vi "options dialog.vi"(9 "mode":string, 10 "Args":T1) -> (1 "mode out":string, 2 "Args out":T1)   [LabVIEW 2016]
uses:
  controls/CL Args.ctl
panel:
  in  "-nobdcosm":bool
  in  "-nobdpos":bool
  in  "DONE":bool
  in  "-nobd":bool
  in  "-nofppos":bool
  in  "-nofp":bool
  in  "-noattr":bool
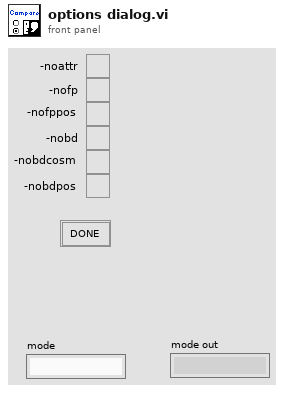
[diagram p1: front panel]
types:
  T1 = typedef "CL Args.ctl" = cluster{"-noattr":bool, "-nofp":bool, "-nofppos":bool, "-nobd":bool, "-nobdcosm":bool, "-nobdpos":bool}
  T2 = enum8{"Enabled", "Disabled", "Disabled and Grayed Out"}
  T3 = enum32{"invalid app kind", "Development System", "Run Time System", "Student Edition", "Embedded LabVIEW", "Evaluation", "Custom"}
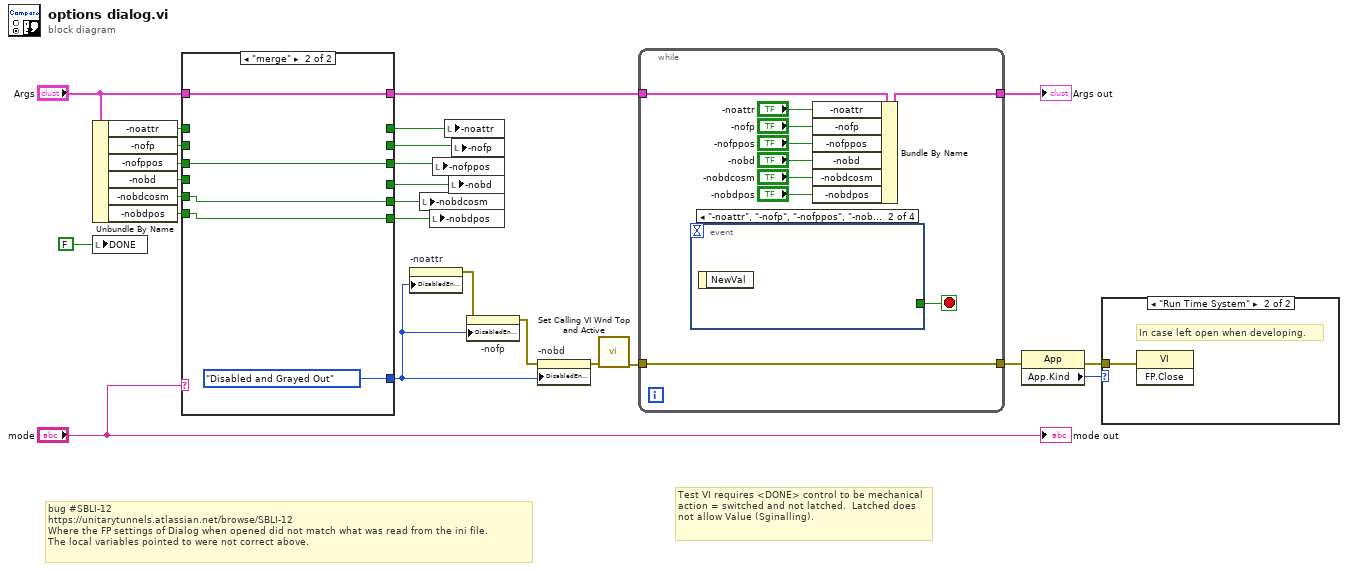
[diagram p0: block diagram]
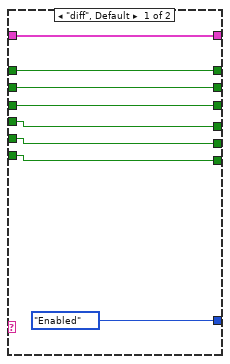
[diagram p2: hidden frame]
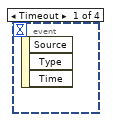
[diagram p4: hidden frame]
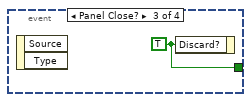
[diagram p5: hidden frame]
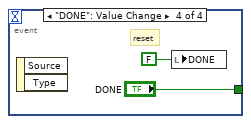
[diagram p6: hidden frame]
diagram:
  # "Test VI requires <DONE> control to be mechanical action = switched and not latched.  Latched does not allow Value (Sginalling)."
  # "bug #SBLI-12 \nhttps://unitarytunnels.atlassian.net/browse/SBLI-12\nWhere the FP settings of Dialog when opened did not match what was read from the ini file.\nThe local variables pointed to were not correct above."
  n1 = Unbundle By Name("Args") -> ("-noattr"=w16:bool, "-nofp"=w15:bool, "-nofppos"=w14:bool, "-nobd"=w13:bool, "-nobdcosm"=w12:bool, "-nobdpos"=w11:bool)
  n2 = local write "DONE"(FALSE ("DONE")) -> ()
  n3 = case shown="\"merge\"" "mode" {
    tunnel: "Args" -> [w33 w38]
    tunnel: [w33 w38] -> w19
    tunnel: [T2."Enabled" ("Disabled") T2."Disabled and Grayed Out" ("Disabled")] -> w18
    tunnel: w16 -> [w31 _]
    tunnel: w15 -> [w30 _]
    tunnel: w14 -> [w29 w36]
    tunnel: w13 -> [w28 _]
    tunnel: w12 -> [w27 w35]
    tunnel: w11 -> [w26 w34]
    tunnel: [w31 _] -> w9
    tunnel: [w30 _] -> w8
    tunnel: [w29 w36] -> w7
    tunnel: [w28 _] -> w6
    tunnel: [w27 w35] -> w5
    tunnel: [w26 w34] -> w4
    frame "diff", Default {
    }
    frame "merge" {
    }
  }
  n4 = property on="-noattr" class="Bool (strict)"("DisabledEnum"=w18) -> (error out=w3:errorcluster)  [unwired: 2 in, 1 out]
  n5 = local write "-nobdcosm"(w5) -> ()
  n6 = local write "-nobdpos"(w4) -> ()
  n7 = local write "-nofppos"(w7) -> ()
  n8 = local write "-noattr"(w9) -> ()
  n9 = local write "-nobd"(w6) -> ()
  n10 = local write "-nofp"(w8) -> ()
  n11 = property on="-nofp" class="Bool (strict)"(error in=w3, "DisabledEnum"=w18) -> (error out=w2:errorcluster)  [unwired: 1 in, 1 out]
  n12 = property on="-nobd" class="Bool (strict)"(error in=w2, "DisabledEnum"=w18) -> (error out=w1:errorcluster)  [unwired: 1 in, 1 out]
  n13 = call "Set Calling VI Wnd Top and Active.vi"("Error In"=w1) -> ("Error Out"=w21:errorcluster)  [unwired: 10 in]
  n14 = while {
    tunnel: [w46] -> w25
    tunnel: w19 -> [w47]
    tunnel: w21 -> [w45]
    tunnel: [w45] -> w23
    stop <- w48 stop-if-true
    n15 = event shown="[1] \"-noattr\", \"-nofp\", \"-nofppos\", \"-nobd\": Value Change" {
      selector: _ -> [_ _ _ _]
      dyn-events: _ -> [_ _ _ _]
      timeout: _ -> [_ _ _ _]
      tunnel: [_ _ w49 "DONE"] -> w48
      event Timeout {
        n16 = event-data() -> ()  [unwired: 1 in, 3 out]
      }
      event "-noattr", "-nofp", "-nofppos", "-nobd": Value Change {
        n17 = event-data() -> ()  [unwired: 1 in, 1 out]
      }
      event Panel Close? {
        w49 = TRUE ("Discard?")
        n18 = event-data() -> ()  [unwired: 1 in, 2 out]
        n19 = event-data("Discard?"=w49) -> ()  [unwired: 1 in, 1 out]
      }
      event "DONE": Value Change {
        # "reset"
        n20 = event-data() -> ()  [unwired: 1 in, 2 out]
        n21 = local write "DONE"(FALSE ("DONE")) -> ()
      }
    }
    n22 = Bundle By Name(cluster=w47, "-noattr"="-noattr", "-nofp"="-nofp", "-nofppos"="-nofppos", "-nobd"="-nobd", "-nobdcosm"="-nobdcosm", "-nobdpos"="-nobdpos") -> (w46:T1)
  }
  "Args out" <- w25
  n23 = property class="App"(error in=w23) -> (error out=w24:errorcluster, "App.Kind"=w22:T3)  [unwired: 1 in, 1 out]
  n24 = case shown="\"Run Time System\"" w22 {
    tunnel: w24 -> [_ w52]
    frame Default {
    }
    frame "Run Time System" {
      # "In case left open when developing."
      n25 = invoke class="VI" method="FP.Close"(error in=w52) -> ()  [unwired: 2 in, 3 out]
    }
  }
  "mode out" <- "mode"
